vi "5492_FlashLED.vi"(0 "x":dbl, 5 "Bank1 Color":u32(colorbox), 7 "Bank2 Color":u32(colorbox), 9 "Bank3 Color":u32(colorbox), 11 "Bank4 Color":u32(colorbox)) -> ()   [LabVIEW 2017]
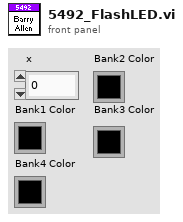
[diagram p1: front panel]
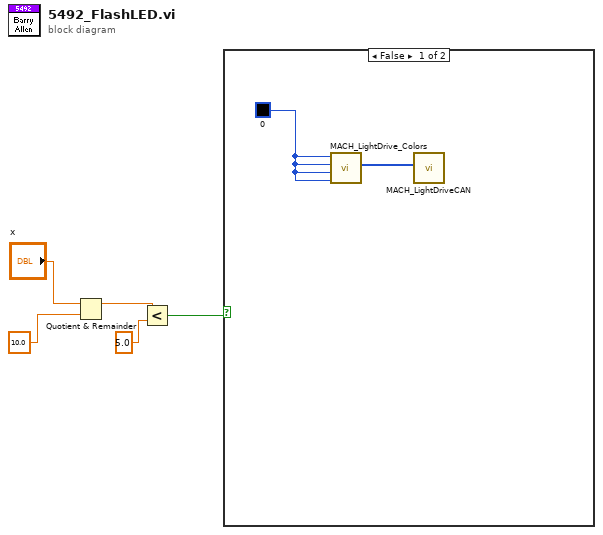
[diagram p0: block diagram]
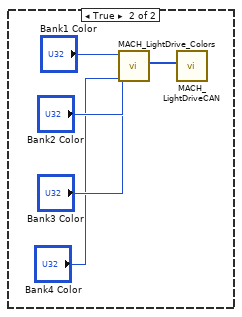
[diagram p2: hidden frame]
diagram:
  n1 = Quotient & Remainder(x="x", y=10.0) -> (x-y*floor(x/y)=w3:dbl)  [unwired: 1 out]
  n2 = Less?(x=w3, y=5.0) -> (x < y?=w1:bool)
  n3 = case shown="False" w1 {
    frame False {
      w6 = u32 0 ("Bank1 Color")
      n4 = call "MACH_LightDrive_Colors.vi"("Bank4 Color"=w6, "Bank3 Color"=w6, "Bank2 Color"=w6, "Bank1 Color"=w6) -> ("Raw Levels"=w7:u8[])  [unwired: 7 in]
      n5 = call "MACH_LightDriveCAN.vi"("Levels"=w7) -> ()  [unwired: 3 in, 8 out]
    }
    frame True {
      n6 = call "MACH_LightDrive_Colors.vi"("Bank4 Color"="Bank4 Color", "Bank3 Color"="Bank3 Color", "Bank2 Color"="Bank2 Color", "Bank1 Color"="Bank1 Color") -> ("Raw Levels"=w12:u8[])  [unwired: 7 in]
      n7 = call "MACH_LightDriveCAN.vi"("Levels"=w12) -> ()  [unwired: 3 in, 8 out]
    }
  }
